vi "Task 3.vi"() -> ()   [LabVIEW 2025]
doc: "Uses two text boxes to demonstrate real-time translation. The user enters English text into Box 1, and upon triggering the translation, the text is sent to the Libre Translate API. The translated German text is then displayed in Box 2."
uses:
  <vilib>/httpClient/POSTBuffer.vi
  <vilib>/httpClient/LabVIEWHTTPClient.lvlib
panel:
  out "German text":string
  in  "English text":string
  in  "Translate":bool
  # "Use 2 text boxes and translate the text inside box1 from English to German into box2 using the API from Libre Translate"
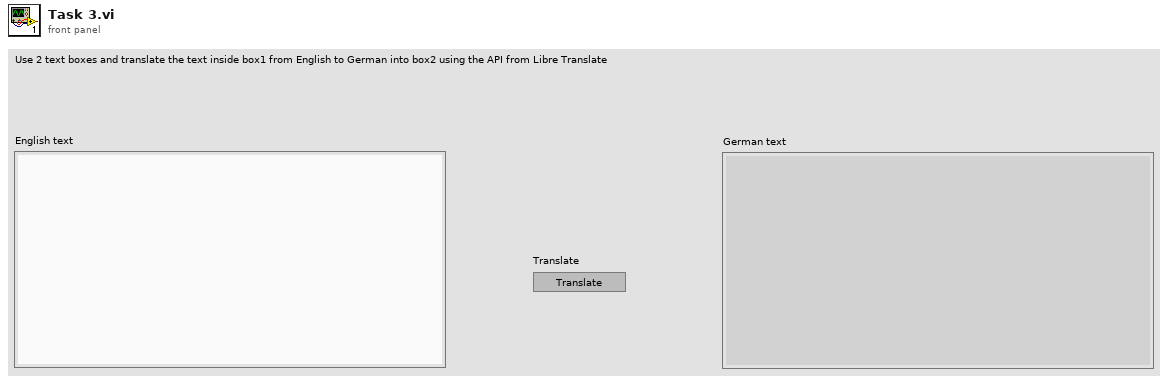
[diagram p1: front panel]
types:
  T1 = typedef "LabVIEWHTTPClient.lvlib/ClientHandle.ctl" = refnum<k1>
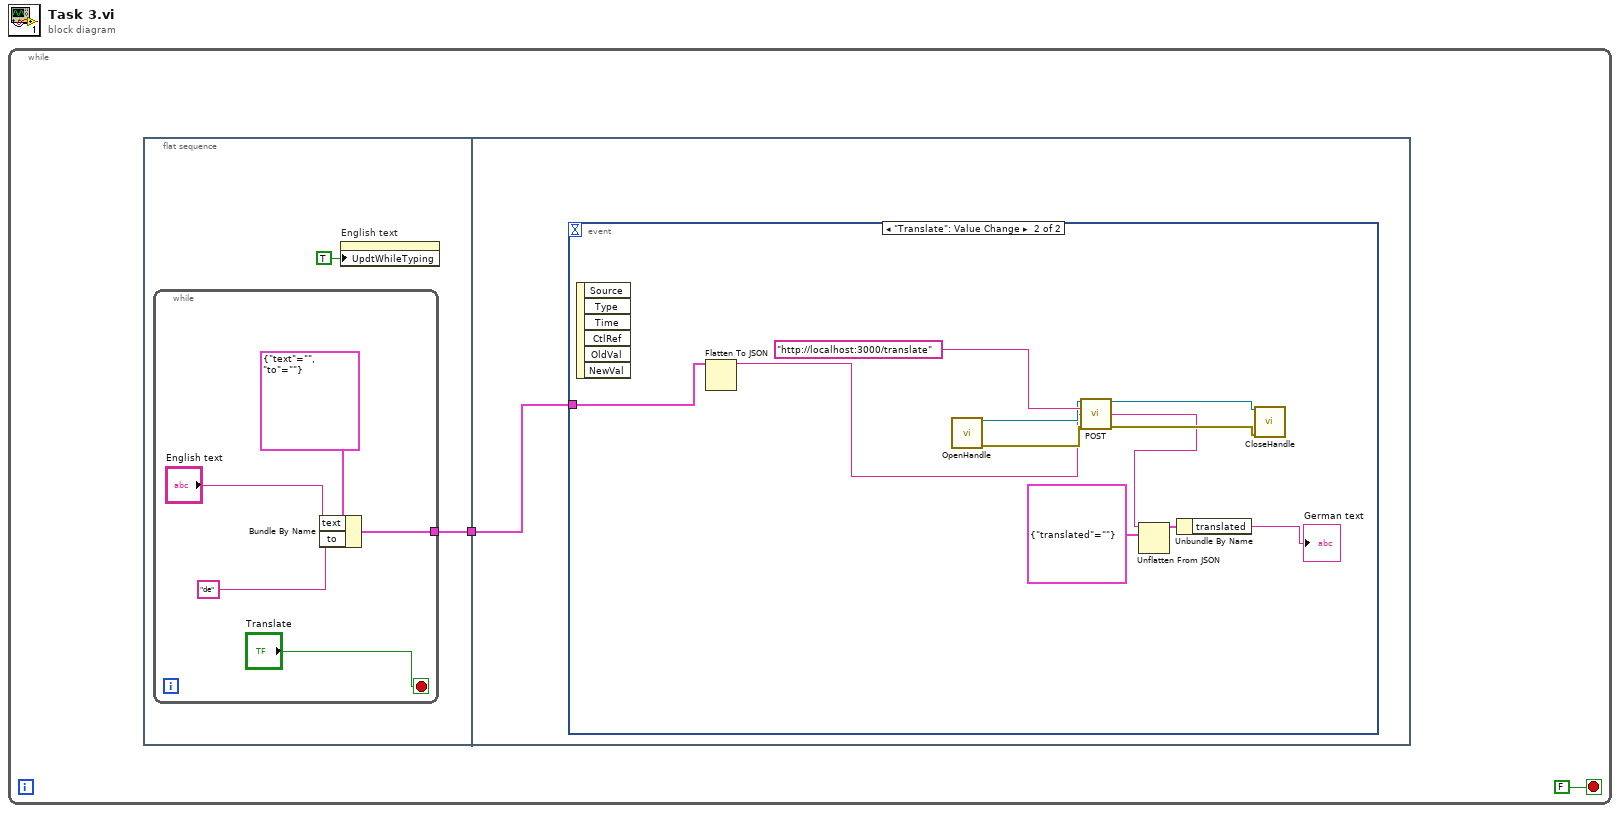
[diagram p0: block diagram]
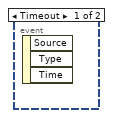
[diagram p2: hidden frame]
diagram:
  n1 = while {
    stop <- FALSE stop-if-true
    n2 = flat-sequence {
      tunnel: [w4] -> w2
      tunnel: w2 -> [w10]
      frame #0 {
        n3 = while {
          tunnel: [w6] -> w4
          stop <- "Translate" stop-if-true
          n4 = Bundle By Name(cluster=cluster{"text":string, "to":string} {"text"="", "to"=""}, "text"="English text", "to"="de") -> (w6:cluster{"text":string, "to":string})
        }
        n5 = property on="English text" class="Str"("UpdtWhileTyping"=TRUE ("Update While Typing?")) -> ()  [unwired: 2 in, 2 out]
      }
      frame #1 {
        n6 = event shown="[1] \"Translate\": Value Change" {
          selector: _ -> [_ _]
          dyn-events: _ -> [_ _]
          timeout: _ -> [_ _]
          tunnel: w10 -> [_ w21]
          event Timeout {
            n7 = event-data() -> ()  [unwired: 1 in, 3 out]
          }
          event "Translate": Value Change {
            n8 = event-data() -> ()  [unwired: 1 in, 6 out]
            n9 = Flatten To JSON(anything=w21) -> (JSON string=w15:string)  [unwired: 2 in, 1 out]
            n10 = call <vilib>:"OpenHandle.vi"() -> ("client handle out"=w18:T1, "error out"=w19:errorcluster)  [unwired: 14 in]
            n11 = call-poly <vilib>:"POST.vi"("client handle"=w18, "url"="http://localhost:3000/translate", "buffer"=w15, "error in (no error)"=w19) -> ("client handle out"=w17:T1, "body"=w12:string, "error out"=w16:errorcluster)  [unwired: 8 in, 1 out]
            n12 = Unflatten From JSON(JSON string=w12, type and defaults=cluster{"translated":string} {"translated"=""}) -> (value=w14:cluster{"translated":string})  [unwired: 5 in, 1 out]
            n13 = Unbundle By Name(w14) -> ("translated"=→"German text":string)
            n14 = call <vilib>:"CloseHandle.vi"("client handle"=w17, "error in (no error)"=w16) -> ()  [unwired: 13 in, 1 out]
          }
        }
      }
    }
  }
